vi "testMap.vi"() -> ()   [LabVIEW 2019, in "AssertionTest.lvlib" / "AssertNotCount.lvlib"]
uses:
  AssertNotCount.lvlib
  Assertion/Assertion.lvlib
panel:
  out "error out":errorcluster
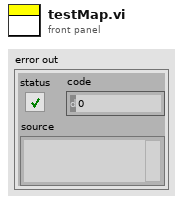
[diagram p1: front panel]
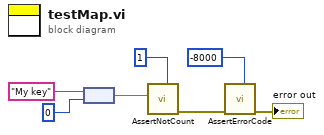
[diagram p0: block diagram]
diagram:
  n1 = node("My key" ("key"), 0 ("value")) -> (w5:map{string, i32})
  n2 = call "AssertNotCount.vi"("Expected"=1, "Haystack"=w5) -> ("error out"=w3:errorcluster)  [unwired: 9 in]
  n3 = call "AssertErrorCode.vi"("Expected"=-8000, "error in (no error)"=w3) -> ("error out"=→"error out":errorcluster)  [unwired: 9 in]
